vi "PvgeneratorOP500P.vi"(8 "errin":errorcluster, 10 "network":path, 11 "path in":path) -> (0 "sortie d'erreur":errorcluster caption="errout", 1 "network out":path, 2 "tout bon":bool, 3 "Chaîne":string)   [LabVIEW 2020]
uses:
  VG/IS30%_P.vi
  VG/VG_OP400_P.vi
  VG/VG_Conti.vi
  VG/VG_ISOmin_P.vi
  VG/VG_TenmaParam.vi
  VG/VG_OCV30min_P.vi
  VG/VG_OCV30max_P.vi
  VG/VG_OCV70min_P.vi
  VG/VG_OCV70max_P.vi
  VG/VG_DCIRmax_P.vi
  VG/VG_DCIRmin_P.vi
  VG/VG_DCIR+OUIouNON_P.vi
panel:
  out "nombre de remplacements":i32
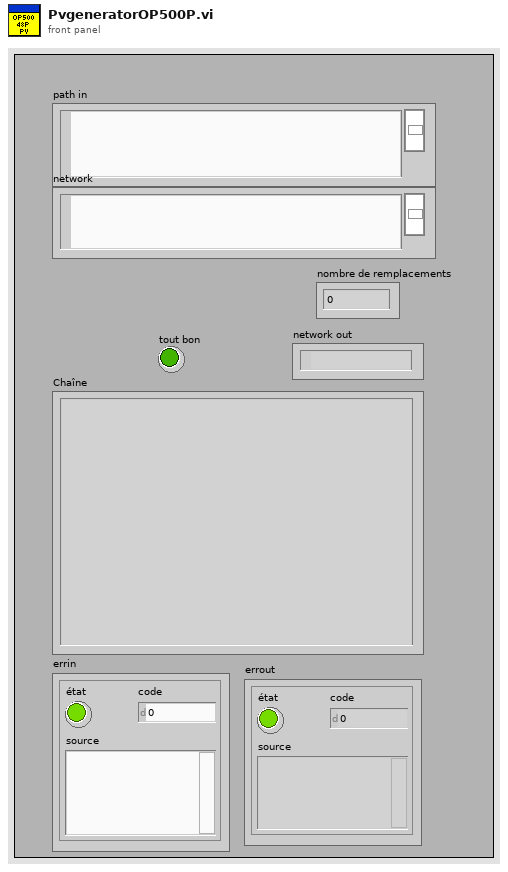
[diagram p1: front panel]
types:
  T1 = enum16{"open", "replace", "create", "open or create", "replace or create", "replace or create with confirmation"}
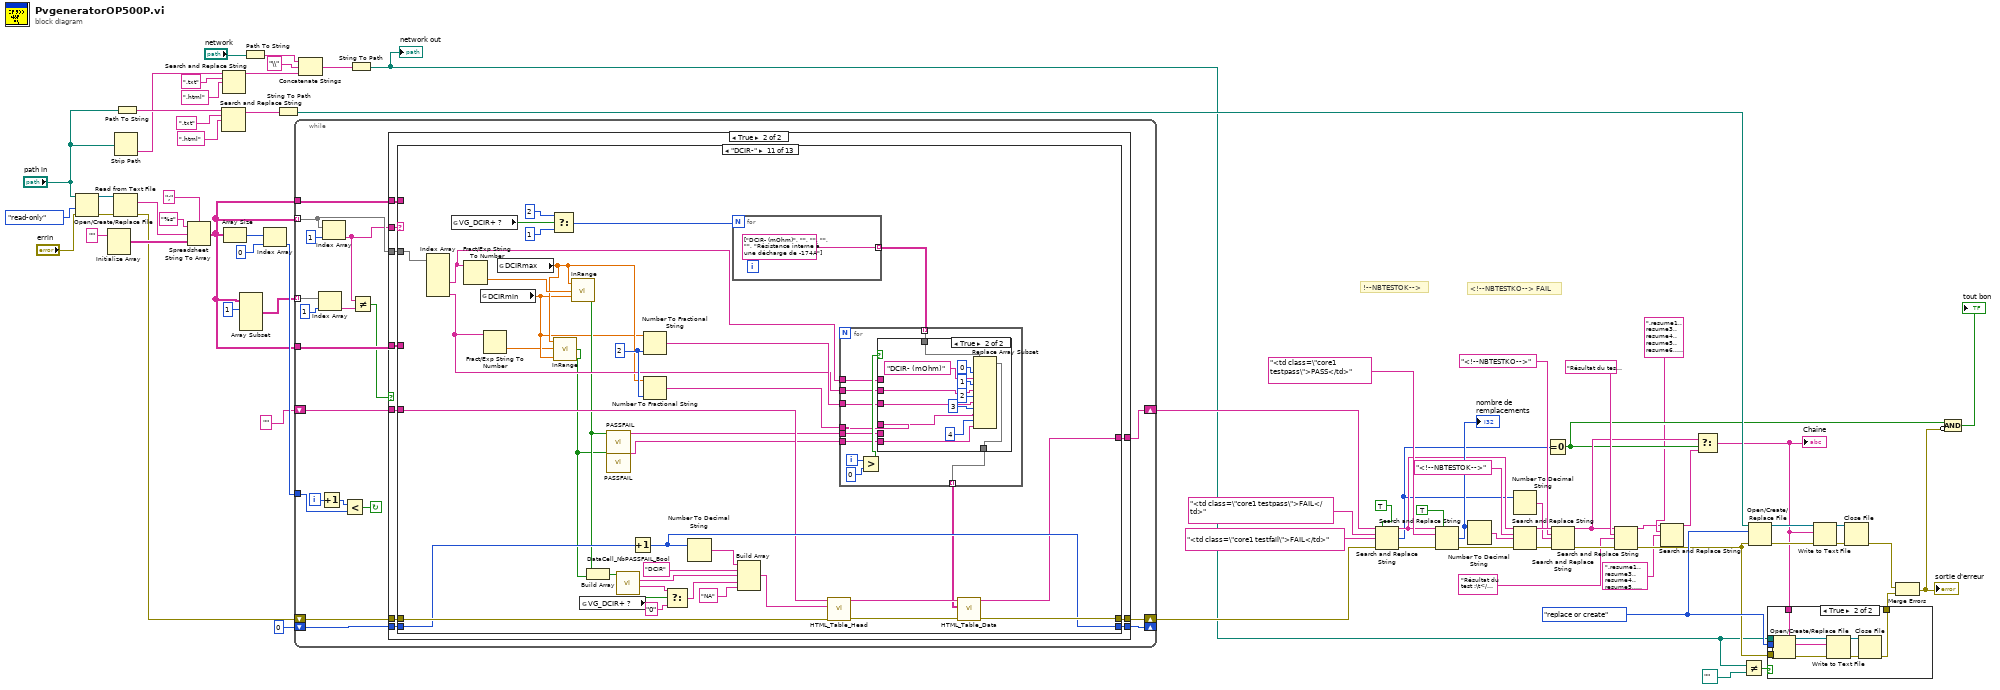
[diagram p0: block diagram]
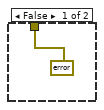
[diagram p2: hidden frame]
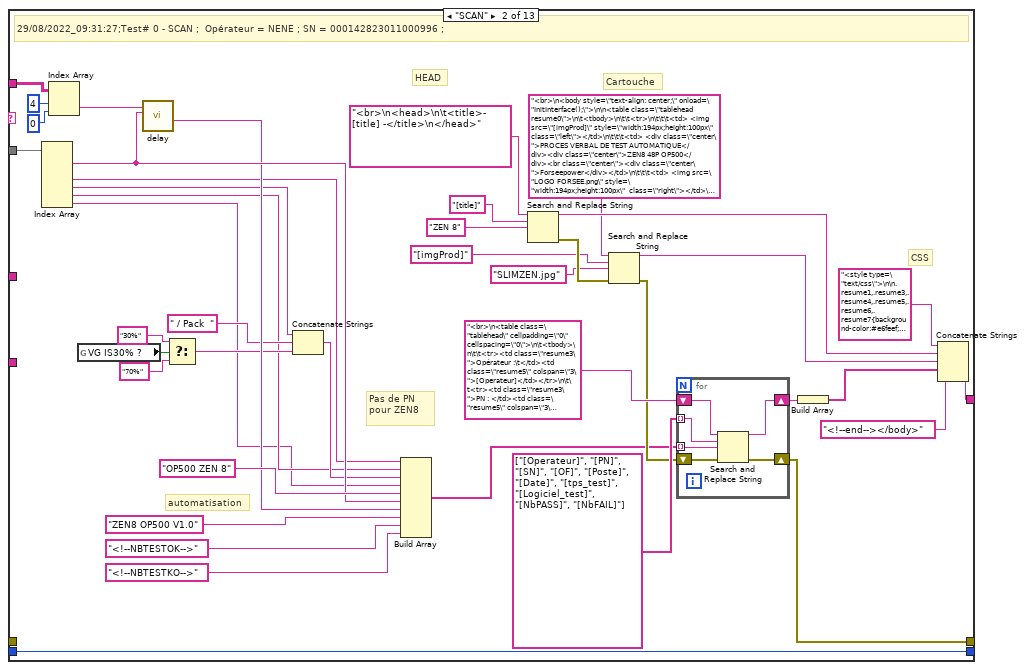
[diagram p5: hidden frame]
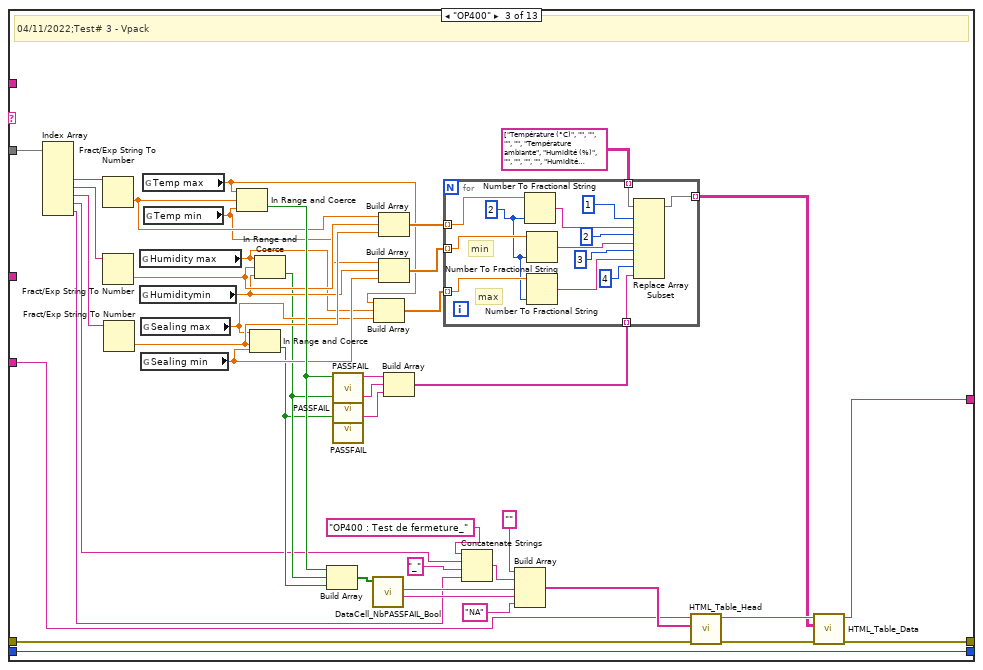
[diagram p6: hidden frame]
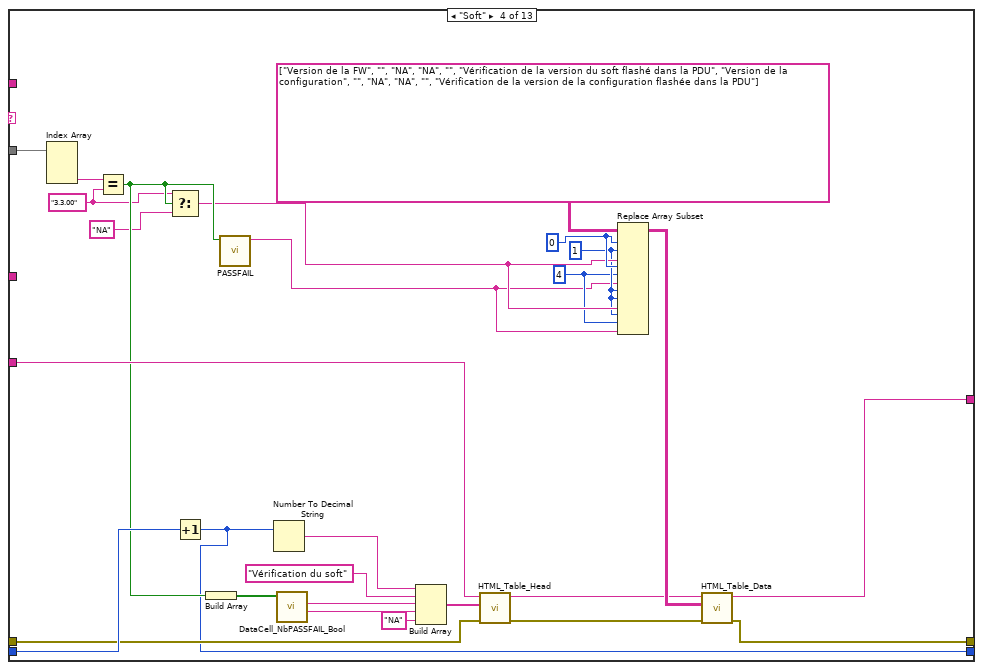
[diagram p7: hidden frame]
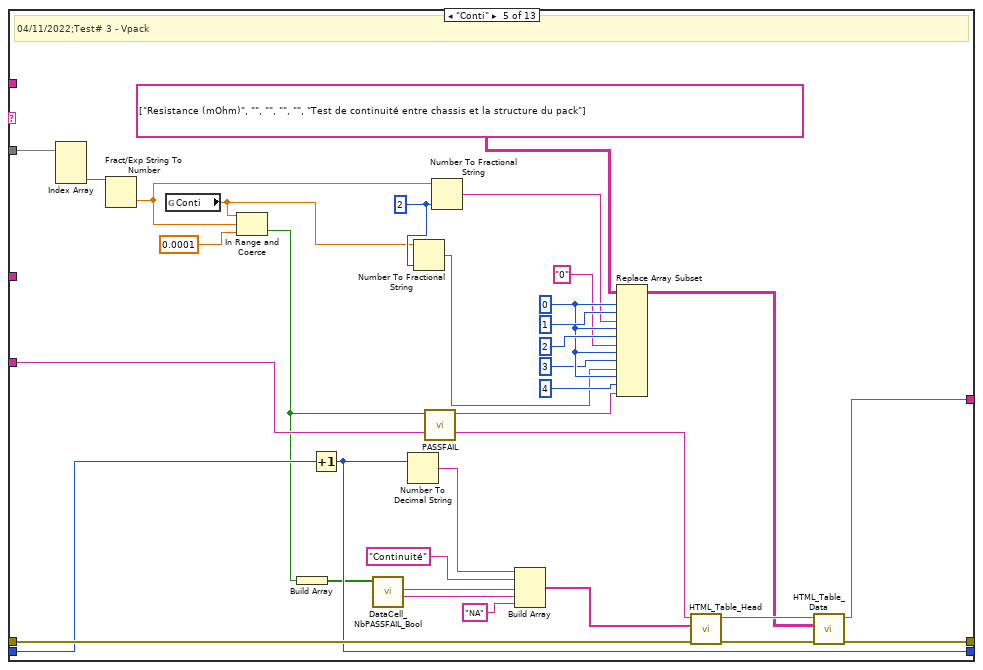
[diagram p8: hidden frame]
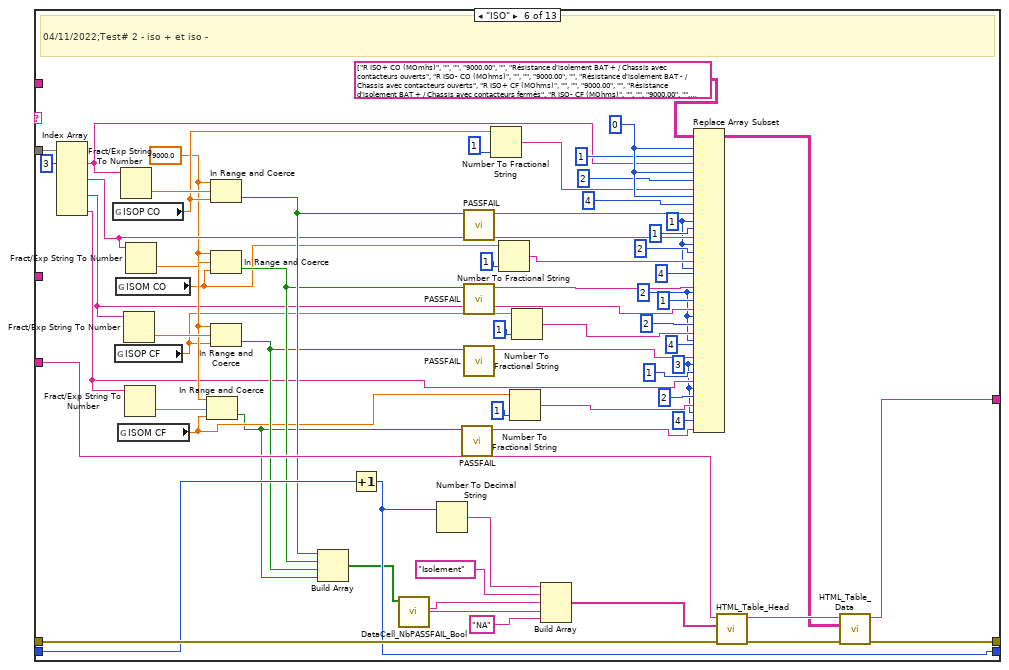
[diagram p9: hidden frame]
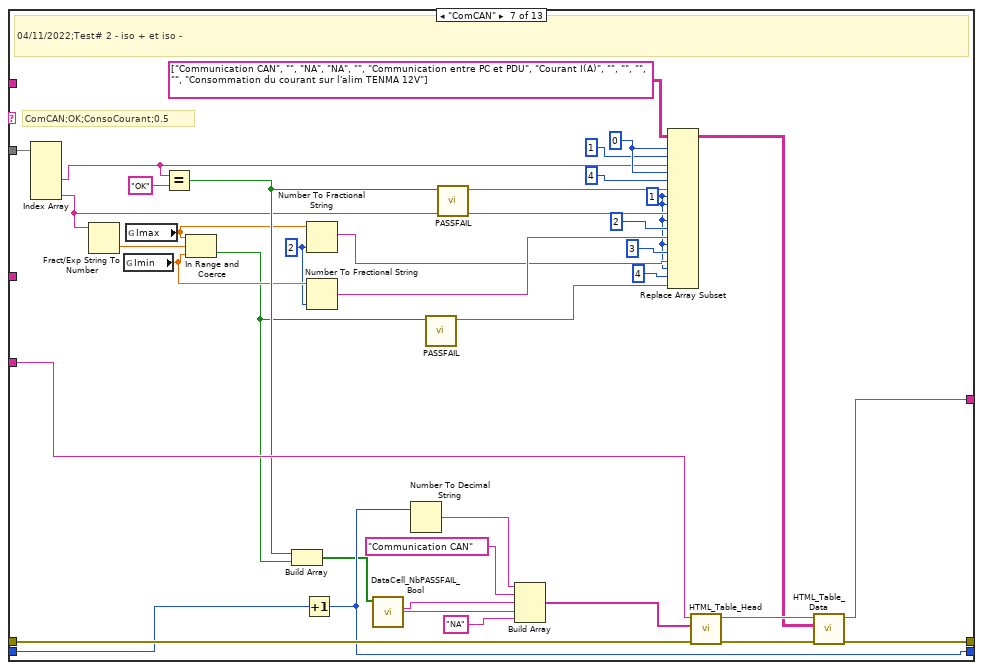
[diagram p10: hidden frame]
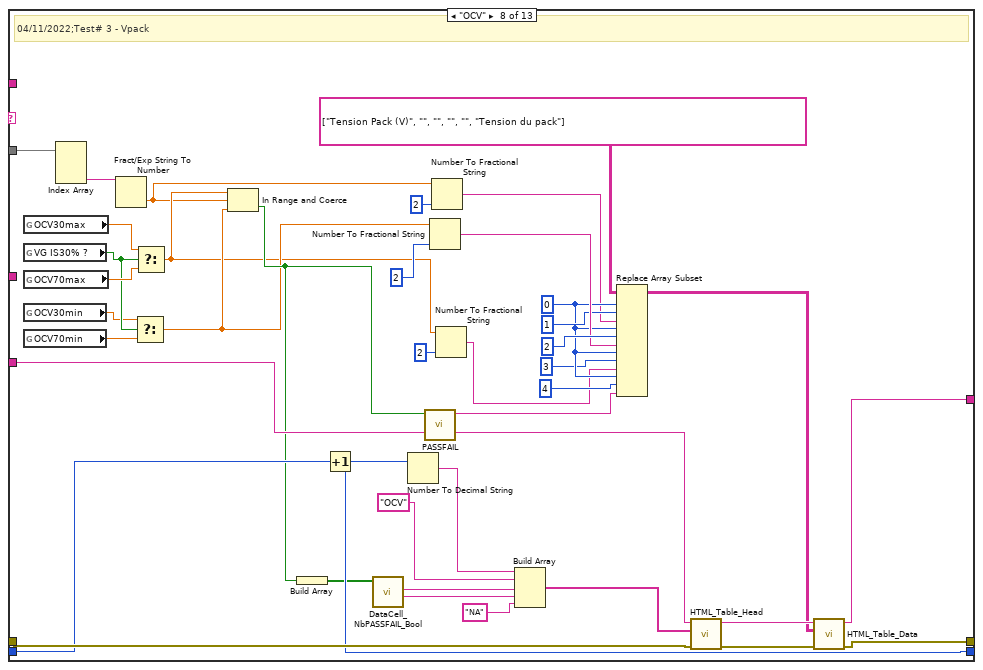
[diagram p11: hidden frame]
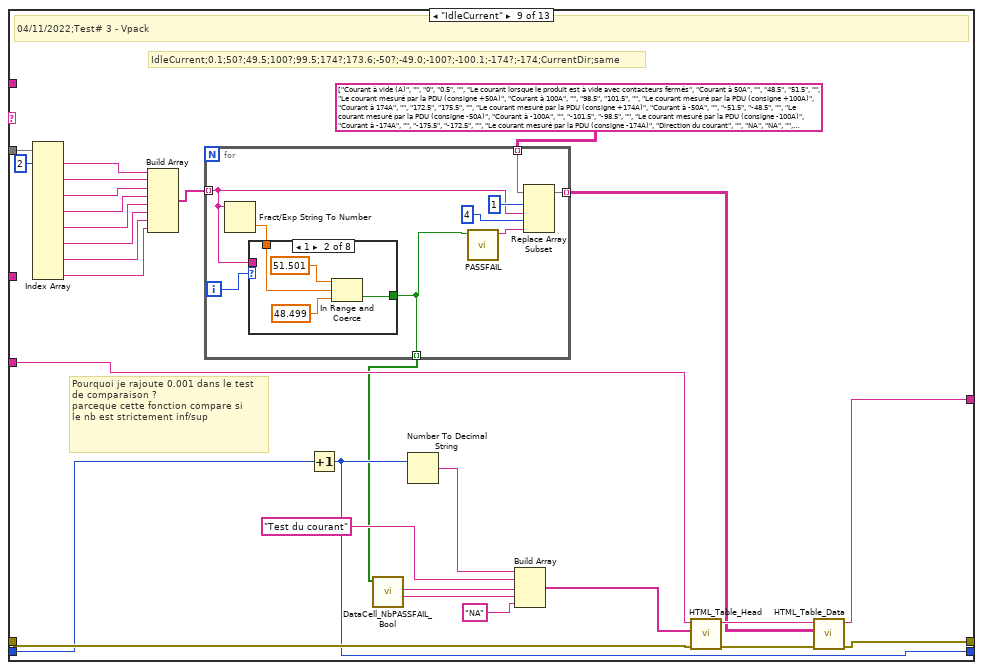
[diagram p12: hidden frame]
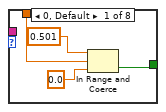
[diagram p13: hidden frame]
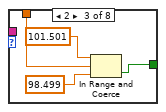
[diagram p14: hidden frame]
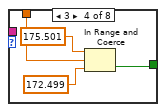
[diagram p15: hidden frame]
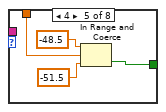
[diagram p16: hidden frame]
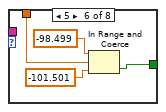
[diagram p17: hidden frame]
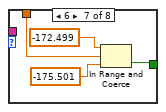
[diagram p18: hidden frame]
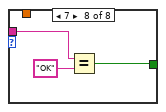
[diagram p19: hidden frame]
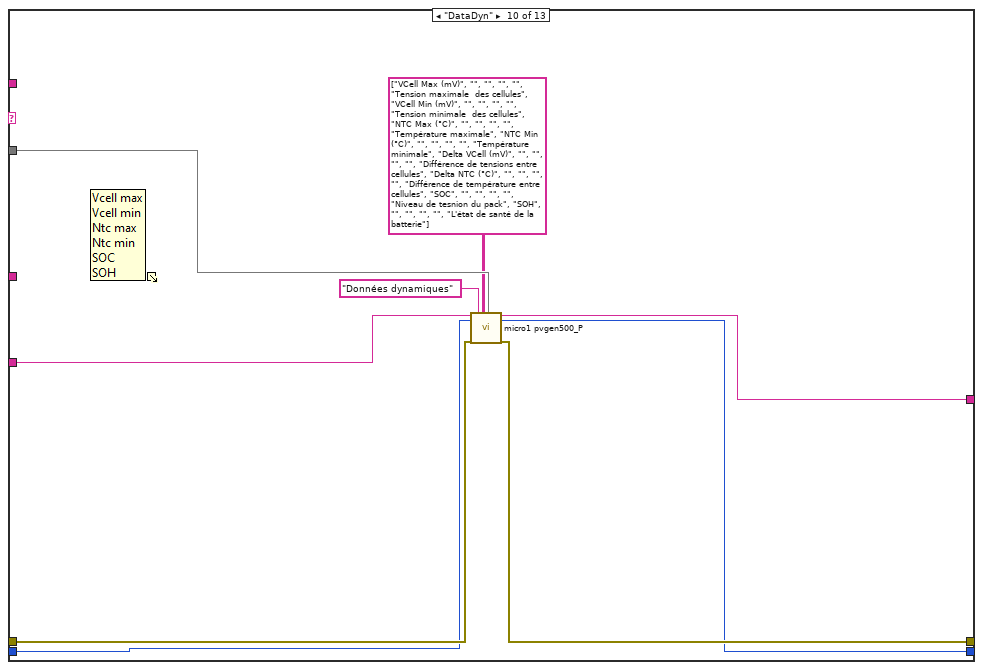
[diagram p20: hidden frame]
diagram:
  w32 = T1."replace or create" ("opération (0 : open)")
  # "<!--NBTESTKO--> FAIL"
  # "!--NBTESTOK-->"
  n1 = Open/Create/Replace File(file path (use dialog)="path in", error in="errin", access (0:read/write)=enum16{"read/write", "read-only", "write-only"}."read-only" ("accès (0 : read/write)")) -> (refnum out=w55:refnum<file>, error out=w72:errorcluster)  [unwired: 3 in, 1 out]
  n2 = Initialize Array("") -> (w70:string[][])  [unwired: 2 in]
  n3 = Read from Text File(file (use dialog)=w55, error in=w72) -> (text=w68:string, error out=w60:errorcluster)  [unwired: 2 in, 2 out]
  n4 = Strip Path(path="path in") -> (name=w13:string)  [unwired: 1 out]
  n5 = Path To String(path="path in") -> (string=w54:string)
  n6 = Spreadsheet String To Array(delimiter (Tab)=";" ("séparateur (Tabulation)"), format string="%s" ("chaîne de format"), spreadsheet string=w68, array type (2D Dbl)=w70) -> (array=w3:string[][])
  n7 = Search and Replace String(input string=w54, search string=".txt" ("chaîne recherchée"), replace string=".html" ("chaîne de remplacement (\"\")")) -> (result string=w51:string)  [unwired: 5 in, 3 out]
  n8 = Search and Replace String(input string=w13, search string=".txt" ("chaîne recherchée"), replace string=".html" ("chaîne de remplacement (\"\")")) -> (result string=w10:string)  [unwired: 5 in, 3 out]
  n9 = Array Size(array=w3) -> (size(s)=w66:i32[])
  n10 = Array Subset(array=w3, index (row)=1 ("indice")) -> (w1:string[][])  [unwired: 3 in]
  n11 = Path To String(path="network") -> (string=w12:string)
  n12 = Index Array(array=w66, index=0 ("indice")) -> (element=w64:i32)
  n13 = String To Path(string=w51) -> (path=w50:path)
  n14 = while {
    tunnel: w64 -> [w91]
    tunnel: w3 -> [w88] mode=indexing
    shift-right: [w87] -> w47
    shift-left: w60 -> [w86]
    shift-right: [w80] -> w49
    shift-left: "" -> [w85]
    shift-right: [w83] -> _
    shift-left: 0 -> [w84]
    tunnel: w3 -> [w82]
    tunnel: w3 -> [w79]
    tunnel: w1 -> [w77] mode=indexing
    i -> [w92]
    stop <- w90 continue-if-true
    n15 = Index Array(array=w77, index=1 ("indice")) -> (element=w76:string)
    n16 = Increment(x=w92) -> (x+1=w81:i32)
    n17 = Index Array(array=w88, index=1 ("indice")) -> (element=w75:string)
    n18 = Less?(x=w81, y=w91) -> (x < y?=w90:bool)
    n19 = Not Equal?(x=w75, y=w76) -> (x != y?=w74:bool)
    n20 = case shown="True" w74 {
      tunnel: w88 -> [_ w105]
      tunnel: [w94 w104] -> w87
      tunnel: w86 -> [w94 w103]
      tunnel: w85 -> [w95 w102]
      tunnel: w84 -> [w93 w101]
      tunnel: [w93 w100] -> w83
      tunnel: w82 -> [_ w99]
      tunnel: [w95 w98] -> w80
      tunnel: w75 -> [_ w97]
      tunnel: w79 -> [_ w96]
      frame False {
      }
      frame True {
        n21 = case shown="\"DCIR-\"" w97 {
          tunnel: w103 -> [w108 _ w192 w234 w264 w328 w366 w406 w435 w491 w525 w589 w618]
          tunnel: w105 -> [_ w149 w193 w228 w265 w329 w367 w407 w436 w487 w528 w579 w608]
          tunnel: [w108 w128 w191 w232 w263 w327 w365 w405 w434 w490 w526 w590 w619] -> w104
          tunnel: w102 -> [w106 _ w190 w238 w262 w326 w364 w404 w433 w485 w519 w580 w609]
          tunnel: w101 -> [w107 w127 w181 w239 w261 w325 w363 w403 w432 w484 w524 w582 w611]
          tunnel: [w107 w127 w181 w214 w260 w324 w362 w402 w431 w483 w521 w564 w603] -> w100
          tunnel: w99 -> [_ _ _ _ _ _ _ _ _ _ _ _ _]
          tunnel: [w106 w126 w189 w216 w259 w323 w361 w401 w430 w489 w512 w578 w607] -> w98
          tunnel: w96 -> [_ w125 _ _ _ _ _ _ _ _ _ _ _]
          frame "NULL", Default {
            # "NULL"
          }
          frame "SCAN" {
            # "automatisation"
            # "Pas de PN pour ZEN8"
            # "Cartouche"
            # "HEAD"
            # "CSS"
            # "29/08/2022_09:31:27;Test# 0 - SCAN ;  Opérateur = NENE ; SN = 000142823011000996 ;"
            n22 = Index Array(array=w149) -> (element #1=w121:string, element #3=w112:string, element #4=w111:string, element #5=w110:string, element #6=w109:string)  [unwired: 6 in, 1 out]
            n23 = Index Array(array=w125, index (row)=4, index (col)=0 ("disabled index (col)")) -> (element=w122:string)
            n24 = global read "IS30%_P.vi" "VG IS30% ?"() -> (w113:bool)
            n25 = call "delay.vi"("String"=w121, "String 2"=w122) -> ("Delay calculé"=w120:string)  [unwired: 9 in]
            n26 = Select(t="30%" ("y"), s=w113, f="70%" ("y")) -> (s? t:f=w116:string)
            n27 = Concatenate Strings(w111, " / Pack  " ("chaîne"), w116) -> (w118:string)
            n28 = Build Array(w112, w110, w118, w109, "OP500 ZEN 8" ("chaîne"), w121, w120, "ZEN8 OP500 V1.0" ("chaîne"), "<!--NBTESTOK-->" ("chaîne"), "<!--NBTESTKO-->" ("chaîne")) -> (w129:string[])
            n29 = Search and Replace String(input string="<br>\n<head>\n\t<title>- [title] -</title>\n</head>", search string="[title]" ("chaîne recherchée"), replace string="ZEN 8" ("Title")) -> (result string=w145:string, error out=w144:errorcluster)  [unwired: 5 in, 2 out]
            n30 = Search and Replace String(input string="<br>\n<body style=\"text-align: center;\" onload=\"InitInterface();\">\n\n<table class=\"tablehead resume0\">\n\t<tbody>\n\t\t<tr>\n\t\t\t<td> <img src=\"[imgProd]\" style=\"width:194px;height:100px\" class=\"left\"></td>\n\t\t\t<td> <div class=\"center\">PROCES VERBAL DE TEST AUTOMATIQUE</div><div class=\"center\">ZEN8 48P OP500</div><br class=\"center\"><div class=\"center\">Forseepower</div></td>\n\t\t\t<td> <img src=\"LOGO FORSEE.png\" style=\"width:194px;height:100px\"  class=\"right\"></td>\n\t\t</tr>\n\t</tbody>\n</table>", search string="[imgProd]", replace string="SLIMZEN.jpg" ("imgProd"), error in=w144) -> (result string=w142:string, error out=w139:errorcluster)  [unwired: 4 in, 2 out]
            n31 = for {
              shift-right: [w154] -> w138
              shift-left: "<br>\n<table class=\"tablehead\" cellpadding=\"0\" cellspacing=\"0\">\n\t<tbody>\n\t\t<tr><td class=\"resume3\">Opérateur :\t</td><td class=\"resume5\" colspan=\"3\">[Operateur]</td></tr>\n\t\t<tr><td class=\"resume3\">PN : </td><td class=\"resume5\" colspan=\"3\">[PN]</td></tr>\n\t\t<tr><td class=\"resume3\">SN : </td><td class=\"resume5\" colspan=\"3\">[SN]</td></tr>\n\t\t<tr><td class=\"resume3\">OF : </td><td class=\"resume5\" colspan=\"3\">[OF]</td></tr>\n\t\t<tr><td class=\"resume3\">Poste : </td><td class=\"resume5\" colspan=\"3\">[Poste]</td></tr>\t\t\n\t\t<tr><td class=\"resume3\">Date du test : </td><td class=\"resume5\" colspan=\"3\">[Date]</td></tr>\n\t\t<tr><td class=\"resume3\">Temps de test : </td><td class=\"resume5\" colspan=\"3\">[tps_test]</td></tr>\n\t\t<tr><td class=\"resume3\">Logiciel de test :\t</td><td class=\"resume5\" colspan=\"3\">[Logiciel_test]</td></tr>\n\t\t<tr><td class=\"resume3\">Résultat du test :\t</td><td class=\"resume5\" colspan=\"3\"><div><span style=\"float:left\" id=\"result\"><font size = \"5pt\" color=\"green\"><b>CONFORME</b></font><b><font size = \"5pt\"> ( </font><font size = \"5pt\" color=\"green\">[NbPASS] PASS </font>  <font size = \"5pt\"> / </font><font size = \"5pt\" color=\"red\">[NbFAIL] FAIL</font> <font size = \"5pt\"> ) </font></b></span></div></td></tr>\n\t</tbody>\n</table>" -> [w155]
              tunnel: string[] ["[Operateur]", "[PN]", "[SN]", "[OF]", "[Poste]", "[Date]", "[tps_test]", "[Logiciel_test]", "[NbPASS]", "[NbFAIL]"] -> [w151] mode=indexing
              tunnel: w129 -> [w150] mode=indexing
              shift-right: [w152] -> w128
              shift-left: w139 -> [w153]
              n32 = Search and Replace String(input string=w155, search string=w151, replace string=w150, error in=w153) -> (result string=w154:string, error out=w152:errorcluster)  [unwired: 4 in, 2 out]
            }
            n33 = Build Array(w138) -> (w137:string[])
            n34 = Concatenate Strings("<style type=\"text/css\">\n\n.resume1,.resume3,.resume4,.resume5,.resume6,.resume7{background-color:#e6feef;padding:7px;border:1px solid black;}\n.resume0{border:1px solid black;background-color:#e6feef;font-weight: bold;padding:0px;text-align: center;}\n.resume1{width:350px;text-align:right;font-weight:bold;}\n.resume3{width:350px;text-align:right;border-top:0px solid black;font-weight:bold;}\n.resume4{border-left:0px solid black;width:290px;}\n.resume5{width:290px;border-left:0px solid black;border-top:0px solid black;}\n.resume6{border-left:0px solid black;width:60px;}\n.resume7{border-left:0px solid black;border-top:0px solid black;width:60px;}\n.title1{text-align: left;background-color:#e6f4fe;padding:10px;border:1px solid #101010;}\n.title2{width: 30px;text-align: center;background-color:#e6f4fe;padding:1px;border:1px solid #101010;border-left:0px solid black;font-weight: bold;}\n.title2 a:link{text-decoration:none;}\n.entete0,.entete1,.entete2,.time2{text-align: center;background-color:#feeec9;padding:7px;border:1px solid black;font-weight: bold;}\n.entete0{width:45px;border-right:0px solid black;}\n.entete1{width:505px;}\n.entete2{width:95px;border-right:0px solid black;}\n.time2{border-left:0px solid black;width:145px;font-size:11px;}\n.core0,.core1,.core2,.core3,.core4,.time{text-align: center;background-color:#fafed3;padding:7px;border:1px solid black;}\n.core0, .core1,.core3,.core4{width:95px;border-top:0px solid black;border-right:0px solid black;}\n.core0{width:45px;}\n.core2{border-top:0px solid black;width:505px;}\n.core3{width:200px;}\n.core4{width:300px;}\n.time{width:145px;border-top:0px solid black;border-left:0px solid black;font-size:11px;}\n.false .core0,.false .core1,.false .core2,.false .core3,.false .core4,.false .time{background-color:#f4f4f4;}\n.false .entete0,.false .entete1,.false .entete2,.false .time2{background-color:#dadada;}\n.false .title1,.false .title2,.false .resultentete .testpass,.false .resultentete .testfail,.false .resultentete .testtime{background-color:#c5cac9;color: blue;}\n.false .title2 a:link{text-decoration:none;color: blue;}\n.comment1,.comment2,.time3{width: 890px;background-color:#e9e8e9;padding:7px;border:1px solid black;border-top:0px solid black;text-align:left;}\n.comment2{border-right:0px solid black;width: 45px;text-align: center;}\n.time3{width: 145px;border-left:0px solid black;font-size:11px;}\n.fixe1{background: -moz-linear-gradient(center top , #101010 10%, #555555 80%) repeat scroll 0 0 transparent;background: -webkit-gradient(linear, left top, left bottom, from(#101010), to(#555555));border:2px solid orange;position : fixed;margin-top:20px;display:none;overflow-y:scroll;max-height:350px;text-shadow: 0px 0px 0 #333333;text-align:left;font-size:10px;padding:10px;margin-left:-162px;border-radius: 15px 15px 15px 15px;}\n.menufixe, .menufixelock{background: -moz-linear-gradient(center top , #101010 80%, transparent 20%) repeat scroll 0 0 transparent;background: -webkit-gradient(linear, left top, left bottom, from(#101010), color-stop(0.65, #101010), to(transparent)) repeat scroll 0 0 transparent;margin: -52px 0px 0px -9px;width:100%;position:fixed;height:55px;-moz-transition: margin 1s;-webkit-transition: margin 1s;}\n.menufixelock, .menufixe:hover{margin: -9px 0px 0px -9px;}\n.lockmenu, .separation,.separationmenu{text-align:center;background: -moz-linear-gradient(center top , #555555 10%, #111111 80%) repeat scroll 0 0 transparent;background: -webkit-gradient(linear, left top, left bottom, from(#555555), to(#111111));border: 1px solid white;border-radius: 10px 10px 10px 10px;box-shadow: 0 -1px 1px #555555 inset;color: #999999;font-weight: bold;width: 100px;padding: 2px;text-decoration: none;}\n.tablehead{width: 1000px;font-family: Verdana;font-size: 12px;margin-left: auto;margin-right: auto;}\n.tablenull{font-family: Verdana;font-size: 11px;margin-left: auto;margin-right: auto;}\n.separationmenu:hover div{display: inline;}\n.lockmenu:hover, .separation:hover,.separationmenu:hover{border: 1px solid orange;cursor:pointer;}\n.lockmenu:hover{border: 1px solid red;cursor:pointer;}\n.separationright{padding:10px;}\ndiv a:link{text-decoration:none;color:#cbcbcb;}\ndiv a:hover{text-decoration:underline;color:#cbcbcb;}\nspan a:link{text-decoration:none;color:#cbcbcb;}\nspan a:hover{text-decoration:none;color:#cbcbcb;}\n.false{color: blue;}\n.testpass{color: green;font-weight: bold;}\n.testfail{color: red;font-weight: bold;}\n.testtime{color: blue;font-weight: bold;}\n.resultentete{font-weight: bold;font-size: 11px;min-width: 200px;text-align:right;}\n.infohard{border: 1px solid black;background-color: white;text-align: center;width: 16px;height: 16px;border-radius: 5px;font-weight: bold;box-shadow: 0 -1px 2px #555555 inset;}\n.infohard:hover{background-color:#feeec9;cursor:pointer;}\n.footerhard{padding-top:30px;}\n.confighard{font-size:10px;width:110px;}\n.circlemain{margin-left:auto;margin-right:auto;}\n.circletext,.circleform{padding-top: 3px;text-align:center;font-size: 10px;width:200px;}\n.circleform{padding-bottom: 3px;padding-top: 1px;}\n.circle{border: 1px solid black;border-collapse: collapse;border-radius: 15px;box-shadow: 1px 1px 0 #505050;height: 15px;width: 15px;display:inline-block;}\n.bookmarkon, .bookmarkoff{background-color: yellow;border: 1px solid black;border-collapse: collapse;border-radius: 10px 10px 10px 10px;box-shadow: 1px 1px 0 #505050;height: 12px;width: 12px;position: absolute;margin-left:22px;cursor: help;}\n.bookmarkoff{background-color: transparent;border: 1px solid #CECECE;box-shadow: none;cursor: copy;}\n.false .bookmarkoff{background-color: transparent;border: 1px solid #E6E1E1;box-shadow: none;cursor: copy;}\n.bookmarkmaster{height: 15px;margin-right: 12px;width: 60px;}\n.bookmarkmaster:hover .bookmarkprev,.bookmarkmaster:hover .bookmarksuiv{display:block;}\n.bookmarkprev, .bookmarksuiv {cursor: pointer;font-size: 25px;font-weight: bold;margin-top: -10px;position: absolute;display:none;}\n.bookmarkprev{margin-left: 2px;}\n.bookmarksuiv{margin-left: 43px;}\n.plus, .moins{background-color: #F4F4F4;border: 1px solid #848484;border-radius: 20px;color: #848484;font-family: arial;font-size: 16px;font-weight: bold;height: 20px;margin-left: 4px;text-align: center;width: 20px;}\n.moins{font-size: 15px;}\n.plus:hover, .moins:hover{background-color: #DADADA;border: 1px solid black;color: black;cursor:pointer;}\n.backtothetop {position: fixed; right: 50%; margin-right: -555px; bottom: 10px; font-size: 35px; font-weight: bold; border: 1px solid #7D7B91; width: 40px; height: 40px; line-height:52px; text-align: center;border-radius: 8px; opacity: 0.25; background-color: #F5F5F5; color:#7D7B91;}\n.backtothetop:hover {opacity: 1; cursor:pointer;}\n.libversion {font-size: 8px;font-weight: normal;padding-right: 10px;text-align: right;}\n.lockmenu {width: 18px;font-size: 12px;}\n.left {display: block; margin-left: 1px;margin-right: auto;}\n.right {display: block; margin-right: 1px;margin-left: auto;}\n.center {display: block; margin-left: auto;margin-right: auto;}\n\n</style>", w145, w142, w137, "<!--end--></body>") -> (w126:string)
          }
          frame "OP400" {
            # "04/11/2022;Test# 3 - Vpack"
            n35 = Index Array(array=w193) -> (element #3=w184:string, element #4=w180:string, element #5=w179:string, element #6=w158:string, element #7=w156:string)  [unwired: 7 in, 2 out]
            n36 = Fract/Exp String To Number(string=w184) -> (number=w178:dbl)  [unwired: 3 in, 1 out]
            n37 = Fract/Exp String To Number(string=w180) -> (number=w177:dbl)  [unwired: 3 in, 1 out]
            n38 = Fract/Exp String To Number(string=w179) -> (number=w176:dbl)  [unwired: 3 in, 1 out]
            n39 = global read "VG_OP400_P.vi" "Humidity max"() -> (w169:dbl)
            n40 = global read "VG_OP400_P.vi" "Humiditymin"() -> (w173:dbl)
            n41 = global read "VG_OP400_P.vi" "Sealing max"() -> (w168:dbl)
            n42 = global read "VG_OP400_P.vi" "Sealing min"() -> (w172:dbl)
            n43 = global read "VG_OP400_P.vi" "Temp max"() -> (w170:dbl)
            n44 = global read "VG_OP400_P.vi" "Temp min"() -> (w174:dbl)
            n45 = In Range and Coerce(upper limit=w170, x=w178, lower limit=w174) -> (In Range?=w183:bool)  [unwired: 1 out]
            n46 = In Range and Coerce(upper limit=w168, x=w176, lower limit=w172) -> (In Range?=w164:bool)  [unwired: 1 out]
            n47 = In Range and Coerce(upper limit=w169, x=w177, lower limit=w173) -> (In Range?=w165:bool)  [unwired: 1 out]
            n48 = Build Array(w183, w165, w164) -> (w187:bool[])
            n49 = call <userlib>:"PASSFAIL.vi"("E"=w183) -> ("S"=w166:string)  [unwired: 10 in]
            n50 = call <userlib>:"PASSFAIL.vi"("E"=w165) -> ("S"=w163:string)  [unwired: 10 in]
            n51 = call <userlib>:"PASSFAIL.vi"("E"=w164) -> ("S"=w162:string)  [unwired: 10 in]
            n52 = call <userlib>:"DataCell_NbPASSFAIL_Bool.vi"("Tableau en entrée"=w187) -> ("Chaîne"=w185:string, "Chaîne 2"=w186:string)  [unwired: 8 in, 1 out]
            n53 = Build Array(w170, w169, w168) -> (w167:dbl[])
            n54 = Build Array(w178, w177, w176) -> (w175:dbl[])
            n55 = Build Array(w174, w173, w172) -> (w171:dbl[])
            n56 = Build Array(w166, w163, w162) -> (w161:string[])
            n57 = for {
              tunnel: string[][] [["Température (°C)", "", "", "", "", "Température ambiante"], ["Humidité (%)", "", "", "", "", "Humidité ambiante"], ["Etanchéité (Pa)", "", "", "", "", "Etanchéité du pack"]] ("Tableau") -> [w212] mode=indexing
              tunnel: [w208] -> w188 mode=indexing
              tunnel: w175 -> [w207] mode=indexing
              tunnel: w171 -> [w204] mode=indexing
              tunnel: w167 -> [w203] mode=indexing
              tunnel: w161 -> [w199] mode=indexing
              w202 = i16 2 ("précision (6)")
              # "max"
              # "min"
              n58 = Number To Fractional String(number=w207, precision (6)=w202) -> (F-format string=w209:string)  [unwired: 2 in]
              n59 = Number To Fractional String(number=w204, precision (6)=w202) -> (F-format string=w210:string)  [unwired: 2 in]
              n60 = Number To Fractional String(number=w203, precision (6)=w202) -> (F-format string=w201:string)  [unwired: 2 in]
              n61 = Replace Array Subset(array=w212, new element #1=w209, index #1=1 ("index"), new element #2=w210, index #2=2 ("index"), new element #3=w201, index #3=3 ("index"), new element #4=w199, index #4=4 ("index")) -> (w208:string[])
            }
            n62 = Concatenate Strings("OP400 : Test de fermeture_" ("élément"), w158, "_" ("string"), w156) -> (w159:string)
            n63 = Build Array("" ("element"), w159, w186, w185, "NA" ("élément")) -> (w197:string[])
            n64 = call "HTML_Table_Head.vi"("entrée d'erreur (pas d'erreur)"=w192, "Tableau"=w197, "chaîne en entrée"=w190) -> ("sortie d'erreur"=w196:errorcluster, "result string"=w195:string)  [unwired: 7 in]
            n65 = call "HTML_Table_Data.vi"("entrée d'erreur (pas d'erreur)"=w196, "Tableau"=w188, "chaîne en entrée"=w195) -> ("sortie d'erreur"=w191:errorcluster, "result string"=w189:string)  [unwired: 7 in]
          }
          frame "Soft" {
            w220 = 4 ("disabled index (col)")
            w223 = 0 ("disabled index (row)")
            w224 = "3.3.00" ("y")
            w221 = 1 ("disabled index (col)")
            n66 = Index Array(array=w228) -> (element #3=w227:string)  [unwired: 3 in, 2 out]
            n67 = Equal?(x=w227, y=w224) -> (x = y?=w225:bool)
            n68 = Select(t=w224, s=w225, f="NA") -> (s? t:f=w222:string)
            n69 = Increment(x=w239) -> (x+1=w214:i32)
            n70 = Build Array(w225) -> (w226:bool[])
            n71 = call <userlib>:"PASSFAIL.vi"("E"=w225) -> ("S"=w219:string)  [unwired: 10 in]
            n72 = Number To Decimal String(number=w214) -> (decimal integer string=w236:string)  [unwired: 1 in]
            n73 = call <userlib>:"DataCell_NbPASSFAIL_Bool.vi"("Tableau en entrée"=w226) -> ("Chaîne"=w230:string, "Chaîne 2"=w231:string)  [unwired: 8 in, 1 out]
            n74 = Build Array(w236, "Vérification du soft" ("element"), w231, w230, "NA" ("element")) -> (w237:string[])
            n75 = call "HTML_Table_Head.vi"("entrée d'erreur (pas d'erreur)"=w234, "Tableau"=w237, "chaîne en entrée"=w238) -> ("sortie d'erreur"=w233:errorcluster, "result string"=w217:string)  [unwired: 7 in]
            n76 = Replace Array Subset(array=string[][] [["Version de la FW", "", "NA", "NA", "", "Vérification de la version du soft flashé dans la PDU"], ["Version de la configuration", "", "NA", "NA", "", "Vérification de la version de la configuration flashée dans la PDU"]] ("Tableau"), new element #1=w222, index (row) #1=w223, index (col) #1=w221, new element #2=w219, index (row) #2=w223, index (col) #2=w220, new element #3=w222, index (row) #3=w221, index (col) #3=w221, new element #4=w219, index (row) #4=w221, index (col) #4=w220) -> (w218:string[][])
            n77 = call "HTML_Table_Data.vi"("entrée d'erreur (pas d'erreur)"=w233, "Tableau"=w218, "chaîne en entrée"=w217) -> ("sortie d'erreur"=w232:errorcluster, "result string"=w216:string)  [unwired: 7 in]
          }
          frame "Conti" {
            w242 = i16 2 ("précision (6)")
            w249 = 0 ("index (row)")
            # "04/11/2022;Test# 3 - Vpack"
            n78 = Index Array(array=w265) -> (element #3=w252:string)  [unwired: 3 in, 2 out]
            n79 = Fract/Exp String To Number(string=w252) -> (number=w246:dbl)  [unwired: 3 in, 1 out]
            n80 = global read "VG_Conti.vi" "Conti"() -> (w241:dbl)
            n81 = In Range and Coerce(upper limit=w241, x=w246, lower limit=0.0001) -> (In Range?=w247:bool)  [unwired: 1 out]
            n82 = Build Array(w247) -> (w257:bool[])
            n83 = Increment(x=w261) -> (x+1=w260:i32)
            n84 = call <userlib>:"DataCell_NbPASSFAIL_Bool.vi"("Tableau en entrée"=w257) -> ("Chaîne"=w255:string, "Chaîne 2"=w256:string)  [unwired: 8 in, 1 out]
            n85 = Number To Decimal String(number=w260) -> (decimal integer string=w268:string)  [unwired: 1 in]
            n86 = Number To Fractional String(number=w241, precision (6)=w242) -> (F-format string=w240:string)  [unwired: 2 in]
            n87 = call <userlib>:"PASSFAIL.vi"("E"=w247) -> ("S"=w251:string)  [unwired: 10 in]
            n88 = Number To Fractional String(number=w246, precision (6)=w242) -> (F-format string=w245:string)  [unwired: 2 in]
            n89 = Build Array(w268, "Continuité" ("élément"), w256, w255, "NA" ("élément")) -> (w271:string[])
            n90 = Replace Array Subset(array=string[][] [["Resistance (mOhm)", "", "", "", "", "Test de continuité entre chassis et la structure du pack"]] ("Tableau"), new element #1=w245, index (row) #1=w249, index (col) #1=1 ("disabled index (col)"), new element #2="0" ("new element/subarray"), index (row) #2=w249, index (col) #2=2 ("disabled index (col)"), new element #3=w240, index (row) #3=w249, index (col) #3=3 ("disabled index (col)"), new element #4=w251, index (row) #4=w249, index (col) #4=4 ("disabled index (col)")) -> (w258:string[][])
            n91 = call "HTML_Table_Head.vi"("entrée d'erreur (pas d'erreur)"=w264, "Tableau"=w271, "chaîne en entrée"=w262) -> ("sortie d'erreur"=w270:errorcluster, "result string"=w269:string)  [unwired: 7 in]
            n92 = call "HTML_Table_Data.vi"("entrée d'erreur (pas d'erreur)"=w270, "Tableau"=w258, "chaîne en entrée"=w269) -> ("sortie d'erreur"=w263:errorcluster, "result string"=w259:string)  [unwired: 7 in]
          }
          frame "ISO" {
            w276 = 3 ("index (row)")
            w284 = 2 ("index (row)")
            w294 = 1 ("index (row)")
            w299 = 9000.0 ("limite supérieure")
            w317 = 0 ("index (row)")
            # "04/11/2022;Test# 2 - iso + et iso -"
            n93 = Index Array(array=w329, index #1=3 ("index")) -> (element #1=w305:string, element #3=w303:string, element #5=w290:string, element #7=w281:string)  [unwired: 6 in, 3 out]
            n94 = global read "VG_ISOmin_P.vi" "ISOP CO"() -> (w307:dbl)
            n95 = global read "VG_ISOmin_P.vi" "ISOP CF"() -> (w288:dbl)
            n96 = global read "VG_ISOmin_P.vi" "ISOM CO"() -> (w296:dbl)
            n97 = global read "VG_ISOmin_P.vi" "ISOM CF"() -> (w278:dbl)
            n98 = Fract/Exp String To Number(string=w305) -> (number=w311:dbl)  [unwired: 3 in, 1 out]
            n99 = Fract/Exp String To Number(string=w290) -> (number=w302:dbl)  [unwired: 3 in, 1 out]
            n100 = Fract/Exp String To Number(string=w281) -> (number=w300:dbl)  [unwired: 3 in, 1 out]
            n101 = Fract/Exp String To Number(string=w303) -> (number=w308:dbl)  [unwired: 3 in, 1 out]
            n102 = In Range and Coerce(upper limit=w299, x=w300, lower limit=w278) -> (In Range?=w273:bool)  [unwired: 1 out]
            n103 = In Range and Coerce(upper limit=w299, x=w311, lower limit=w307) -> (In Range?=w310:bool)  [unwired: 1 out]
            n104 = In Range and Coerce(upper limit=w299, x=w308, lower limit=w296) -> (In Range?=w309:bool)  [unwired: 1 out]
            n105 = In Range and Coerce(upper limit=w299, x=w302, lower limit=w288) -> (In Range?=w301:bool)  [unwired: 1 out]
            n106 = Build Array(w310, w309, w301, w273) -> (w321:bool[])
            n107 = Increment(x=w325) -> (x+1=w324:i32)
            n108 = call <userlib>:"DataCell_NbPASSFAIL_Bool.vi"("Tableau en entrée"=w321) -> ("Chaîne"=w319:string, "Chaîne 2"=w320:string)  [unwired: 8 in, 1 out]
            n109 = Number To Decimal String(number=w324) -> (decimal integer string=w332:string)  [unwired: 1 in]
            n110 = call <userlib>:"PASSFAIL.vi"("E"=w273) -> ("S"=w274:string)  [unwired: 10 in]
            n111 = call <userlib>:"PASSFAIL.vi"("E"=w310) -> ("S"=w316:string)  [unwired: 10 in]
            n112 = call <userlib>:"PASSFAIL.vi"("E"=w309) -> ("S"=w292:string)  [unwired: 10 in]
            n113 = call <userlib>:"PASSFAIL.vi"("E"=w301) -> ("S"=w283:string)  [unwired: 10 in]
            n114 = Number To Fractional String(number=w307, precision (6)=i16 1) -> (F-format string=w312:string)  [unwired: 2 in]
            n115 = Number To Fractional String(number=w296, precision (6)=i16 1) -> (F-format string=w295:string)  [unwired: 2 in]
            n116 = Number To Fractional String(number=w278, precision (6)=i16 1) -> (F-format string=w277:string)  [unwired: 2 in]
            n117 = Number To Fractional String(number=w288, precision (6)=i16 1) -> (F-format string=w287:string)  [unwired: 2 in]
            n118 = Build Array(w332, "Isolement" ("élément"), w320, w319, "NA" ("élément")) -> (w335:string[])
            n119 = Replace Array Subset(array=string[][] [["R ISO+ CO (MOmhs)", "", "", "9000.00", "", "Résistance d'isolement BAT + / Chassis avec contacteurs ouverts"], ["R ISO- CO (MOhms)", "", "", "9000.00", "", "Résistance d'isolement BAT - / Chassis avec contacteurs ouverts"], ["R ISO+ CF (MOhms)", "", "", "9000.00", "", "Résistance d'isolement BAT + / Chassis avec contacteurs fermés"], ["R ISO- CF (MOhms)", "", "", "9000.00", "", "Résistance d'isolement BAT - / Chassis avec contacteurs fermés"]] ("Tableau"), new element #1=w305, index (row) #1=w317, index (col) #1=1 ("disabled index (col)"), new element #2=w312, index (row) #2=w317, index (col) #2=2 ("disabled index (col)"), new element #3=w316, index (row) #3=w317, index (col) #3=4 ("disabled index (col)"), new element #4=w303, index (row) #4=w294, index (col) #4=1 ("disabled index (col)"), new element #5=w295, index (row) #5=w294, index (col) #5=2 ("disabled index (col)"), new element #6=w292, index (row) #6=w294, index (col) #6=4 ("disabled index (col)"), new element #7=w290, index (row) #7=w284, index (col) #7=1 ("disabled index (col)"), new element #8=w287, index (row) #8=w284, index (col) #8=2 ("disabled index (col)"), new element #9=w283, index (row) #9=w284, index (col) #9=4 ("index (row)"), new element #10=w281, index (row) #10=w276, index (col) #10=1 ("disabled index (col)"), new element #11=w277, index (row) #11=w276, index (col) #11=2 ("disabled index (col)"), new element #12=w274, index (row) #12=w276, index (col) #12=4 ("disabled index (col)")) -> (w322:string[][])
            n120 = call "HTML_Table_Head.vi"("entrée d'erreur (pas d'erreur)"=w328, "Tableau"=w335, "chaîne en entrée"=w326) -> ("sortie d'erreur"=w334:errorcluster, "result string"=w333:string)  [unwired: 7 in]
            n121 = call "HTML_Table_Data.vi"("entrée d'erreur (pas d'erreur)"=w334, "Tableau"=w322, "chaîne en entrée"=w333) -> ("sortie d'erreur"=w327:errorcluster, "result string"=w323:string)  [unwired: 7 in]
          }
          frame "ComCAN" {
            w337 = i16 2 ("precision (6)")
            w340 = 1 ("index (row)")
            w356 = 0 ("index (row)")
            # "ComCAN;OK;ConsoCourant;0.5"
            # "04/11/2022;Test# 2 - iso + et iso -"
            n122 = Index Array(array=w367) -> (element #3=w351:string, element #5=w348:string)  [unwired: 5 in, 3 out]
            n123 = Fract/Exp String To Number(string=w348) -> (number=w353:dbl)  [unwired: 3 in, 1 out]
            n124 = global read "VG_TenmaParam.vi" "Imin"() -> (w346:dbl)
            n125 = global read "VG_TenmaParam.vi" "Imax"() -> (w347:dbl)
            n126 = Equal?(x=w351, y="OK") -> (x = y?=w349:bool)
            n127 = In Range and Coerce(upper limit=w347, x=w353, lower limit=w346) -> (In Range?=w341:bool)  [unwired: 1 out]
            n128 = Build Array(w349, w341) -> (w359:bool[])
            n129 = Increment(x=w363) -> (x+1=w362:i32)
            n130 = Number To Fractional String(number=w347, precision (6)=w337) -> (F-format string=w342:string)  [unwired: 2 in]
            n131 = Number To Fractional String(number=w346, precision (6)=w337) -> (F-format string=w344:string)  [unwired: 2 in]
            n132 = call <userlib>:"DataCell_NbPASSFAIL_Bool.vi"("Tableau en entrée"=w359) -> ("Chaîne"=w357:string, "Chaîne 2"=w358:string)  [unwired: 8 in, 1 out]
            n133 = Number To Decimal String(number=w362) -> (decimal integer string=w370:string)  [unwired: 1 in]
            n134 = call <userlib>:"PASSFAIL.vi"("E"=w341) -> ("S"=w338:string)  [unwired: 10 in]
            n135 = call <userlib>:"PASSFAIL.vi"("E"=w349) -> ("S"=w352:string)  [unwired: 10 in]
            n136 = Build Array(w370, "Communication CAN" ("élément"), w358, w357, "NA" ("élément")) -> (w373:string[])
            n137 = Replace Array Subset(array=string[][] [["Communication CAN", "", "NA", "NA", "", "Communication entre PC et PDU"], ["Courant I(A)", "", "", "", "", "Consommation du courant sur l'alim TENMA 12V"]] ("Tableau"), new element #1=w351, index (row) #1=w356, index (col) #1=1 ("disabled index (col)"), new element #2=w352, index (row) #2=w356, index (col) #2=4 ("disabled index (col)"), new element #3=w348, index (row) #3=w340, index (col) #3=w340, new element #4=w344, index (row) #4=w340, index (col) #4=2 ("disabled index (col)"), new element #5=w342, index (row) #5=w340, index (col) #5=3 ("disabled index (col)"), new element #6=w338, index (row) #6=w340, index (col) #6=4 ("disabled index (col)")) -> (w360:string[][])
            n138 = call "HTML_Table_Head.vi"("entrée d'erreur (pas d'erreur)"=w366, "Tableau"=w373, "chaîne en entrée"=w364) -> ("sortie d'erreur"=w372:errorcluster, "result string"=w371:string)  [unwired: 7 in]
            n139 = call "HTML_Table_Data.vi"("entrée d'erreur (pas d'erreur)"=w372, "Tableau"=w360, "chaîne en entrée"=w371) -> ("sortie d'erreur"=w365:errorcluster, "result string"=w361:string)  [unwired: 7 in]
          }
          frame "OCV" {
            w389 = 0 ("index (row)")
            # "04/11/2022;Test# 3 - Vpack"
            n140 = global read "VG_OCV30max_P.vi" "OCV30max"() -> (w384:dbl)
            n141 = global read "IS30%_P.vi" "VG IS30% ?"() -> (w382:bool)
            n142 = global read "VG_OCV70max_P.vi" "OCV70max"() -> (w383:dbl)
            n143 = global read "VG_OCV30min_P.vi" "OCV30min"() -> (w381:dbl)
            n144 = global read "VG_OCV70min_P.vi" "OCV70min"() -> (w380:dbl)
            n145 = Index Array(array=w407) -> (element #3=w392:string)  [unwired: 3 in, 2 out]
            n146 = Fract/Exp String To Number(string=w392) -> (number=w377:dbl)  [unwired: 3 in, 1 out]
            n147 = Select(t=w381, s=w382, f=w380) -> (s? t:f=w379:dbl)
            n148 = Select(t=w384, s=w382, f=w383) -> (s? t:f=w378:dbl)
            n149 = In Range and Coerce(upper limit=w378, x=w377, lower limit=w379) -> (In Range?=w387:bool)  [unwired: 1 out]
            n150 = Build Array(w387) -> (w399:bool[])
            n151 = Increment(x=w403) -> (x+1=w402:i32)
            n152 = call <userlib>:"DataCell_NbPASSFAIL_Bool.vi"("Tableau en entrée"=w399) -> ("Chaîne"=w397:string, "Chaîne 2"=w398:string)  [unwired: 8 in, 1 out]
            n153 = Number To Decimal String(number=w402) -> (decimal integer string=w410:string)  [unwired: 1 in]
            n154 = call <userlib>:"PASSFAIL.vi"("E"=w387) -> ("S"=w391:string)  [unwired: 10 in]
            n155 = Number To Fractional String(number=w379, precision (6)=i16 2) -> (F-format string=w395:string)  [unwired: 2 in]
            n156 = Number To Fractional String(number=w377, precision (6)=i16 2 ("précision (6)")) -> (F-format string=w376:string)  [unwired: 2 in]
            n157 = Number To Fractional String(number=w378, precision (6)=i16 2) -> (F-format string=w385:string)  [unwired: 2 in]
            n158 = Build Array(w410, "OCV" ("élément"), w398, w397, "NA" ("élément")) -> (w413:string[])
            n159 = Replace Array Subset(array=string[][] [["Tension Pack (V)", "", "", "", "", "Tension du pack"]] ("Tableau"), new element #1=w376, index (row) #1=w389, index (col) #1=1 ("disabled index (col)"), new element #2=w395, index (row) #2=w389, index (col) #2=2 ("disabled index (col)"), new element #3=w385, index (row) #3=w389, index (col) #3=3 ("disabled index (col)"), new element #4=w391, index (row) #4=w389, index (col) #4=4 ("disabled index (col)")) -> (w400:string[][])
            n160 = call "HTML_Table_Head.vi"("entrée d'erreur (pas d'erreur)"=w406, "Tableau"=w413, "chaîne en entrée"=w404) -> ("sortie d'erreur"=w412:errorcluster, "result string"=w411:string)  [unwired: 7 in]
            n161 = call "HTML_Table_Data.vi"("entrée d'erreur (pas d'erreur)"=w412, "Tableau"=w400, "chaîne en entrée"=w411) -> ("sortie d'erreur"=w405:errorcluster, "result string"=w401:string)  [unwired: 7 in]
          }
          frame "IdleCurrent" {
            # "Pourquoi je rajoute 0.001 dans le test \nde comparaison ?\nparceque cette fonction compare si \nle nb est strictement inf/sup"
            # "IdleCurrent;0.1;50?;49.5;100?;99.5;174?;173.6;-50?;-49.0;-100?;-100.1;-174?;-174;CurrentDir;same"
            # "04/11/2022;Test# 3 - Vpack"
            n162 = Index Array(array=w436, index #1=2 ("index")) -> (element #1=w425:string, element #3=w424:string, element #5=w423:string, element #7=w422:string, element #9=w421:string, element #11=w420:string, element #13=w419:string, element #15=w418:string)  [unwired: 14 in, 7 out]
            n163 = Build Array(w425, w424, w423, w422, w421, w420, w419, w418) -> (w417:string[])
            n164 = for {
              tunnel: string[][] [["Courant à vide (A)", "", "0", "0.5", "", "Le courant lorsque le produit est à vide avec contacteurs fermés"], ["Courant à 50A", "", "48.5", "51.5", "", "Le courant mesuré par la PDU (consigne +50A)"], ["Courant à 100A", "", "98.5", "101.5", "", "Le courant mesuré par la PDU (consigne +100A)"], ["Courant à 174A", "", "172.5", "175.5", "", "Le courant mesuré par la PDU (consigne +174A)"], ["Courant à -50A", "", "-51.5", "-48.5", "", "Le courant mesuré par la PDU (consigne -50A)"], ["Courant à -100A", "", "-101.5", "-98.5", "", "Le courant mesuré par la PDU (consigne -100A)"], ["Courant à -174A", "", "-175.5", "-172.5", "", "Le courant mesuré par la PDU (consigne -174A)"], ["Direction du courant", "", "NA", "NA", "", "Verification du sens du courant entre la PDU est l'alimentaion ITECH"]] ("Tableau") -> [w451] mode=indexing
              tunnel: w417 -> [w445] mode=indexing
              tunnel: [w444] -> w426 mode=indexing
              tunnel: [w443] -> w416 mode=indexing
              i -> [w448]
              n165 = Fract/Exp String To Number(string=w445) -> (number=w446:dbl)  [unwired: 3 in, 1 out]
              n166 = case shown="1" w448 {
                tunnel: [w455 w459 w463 w464 w468 w472 w479 w480] -> w443
                tunnel: w446 -> [w452 w456 w460 w465 w469 w473 w476 _]
                tunnel: w445 -> [_ _ _ _ _ _ _ w482]
                frame 0, Default {
                  n167 = In Range and Coerce(upper limit=0.501, x=w452, lower limit=0.0 ("upper limit")) -> (In Range?=w455:bool)  [unwired: 1 out]
                }
                frame 1 {
                  n168 = In Range and Coerce(upper limit=51.501, x=w456, lower limit=48.499 ("upper limit")) -> (In Range?=w459:bool)  [unwired: 1 out]
                }
                frame 2 {
                  n169 = In Range and Coerce(upper limit=101.501, x=w460, lower limit=98.499 ("upper limit")) -> (In Range?=w463:bool)  [unwired: 1 out]
                }
                frame 3 {
                  n170 = In Range and Coerce(upper limit=175.501, x=w465, lower limit=172.499 ("upper limit")) -> (In Range?=w464:bool)  [unwired: 1 out]
                }
                frame 4 {
                  n171 = In Range and Coerce(upper limit=-48.5, x=w469, lower limit=-51.5 ("upper limit")) -> (In Range?=w468:bool)  [unwired: 1 out]
                }
                frame 5 {
                  n172 = In Range and Coerce(upper limit=-98.499, x=w473, lower limit=-101.501 ("upper limit")) -> (In Range?=w472:bool)  [unwired: 1 out]
                }
                frame 6 {
                  n173 = In Range and Coerce(upper limit=-172.499, x=w476, lower limit=-175.501 ("upper limit")) -> (In Range?=w479:bool)  [unwired: 1 out]
                }
                frame 7 {
                  n174 = Equal?(x=w482, y="OK") -> (x = y?=w480:bool)
                }
              }
              n175 = call <userlib>:"PASSFAIL.vi"("E"=w443) -> ("S"=w447:string)  [unwired: 10 in]
              n176 = Replace Array Subset(array=w451, new element #1=w445, index #1=1 ("index"), new element #2=w447, index #2=4 ("index")) -> (w444:string[])
            }
            n177 = Increment(x=w432) -> (x+1=w431:i32)
            n178 = call <userlib>:"DataCell_NbPASSFAIL_Bool.vi"("Tableau en entrée"=w416) -> ("Chaîne"=w428:string, "Chaîne 2"=w429:string)  [unwired: 8 in, 1 out]
            n179 = Number To Decimal String(number=w431) -> (decimal integer string=w439:string)  [unwired: 1 in]
            n180 = Build Array(w439, "Test du courant" ("élément"), w429, w428, "NA" ("élément")) -> (w442:string[])
            n181 = call "HTML_Table_Head.vi"("entrée d'erreur (pas d'erreur)"=w435, "Tableau"=w442, "chaîne en entrée"=w433) -> ("sortie d'erreur"=w441:errorcluster, "result string"=w440:string)  [unwired: 7 in]
            n182 = call "HTML_Table_Data.vi"("entrée d'erreur (pas d'erreur)"=w441, "Tableau"=w426, "chaîne en entrée"=w440) -> ("sortie d'erreur"=w434:errorcluster, "result string"=w430:string)  [unwired: 7 in]
          }
          frame "DataDyn" {
            n183 = call "micro1 pvgen500_P.vi"("FluxStrIn"=w485, "Numin"=w484, "errin"=w491, "Data label"="Données dynamiques" ("testlabel"), "tab ref"=string[][] [["VCell Max (mV)", "", "", "", "", "Tension maximale  des cellules"], ["VCell Min (mV)", "", "", "", "", "Tension minimale  des cellules"], ["NTC Max (°C)", "", "", "", "", "Température maximale"], ["NTC Min (°C)", "", "", "", "", "Température minimale"], ["Delta VCell (mV)", "", "", "", "", "Différence de tensions entre cellules"], ["Delta NTC (°C)", "", "", "", "", "Différence de température entre cellules"], ["SOC", "", "", "", "", "Niveau de tesnion du pack"], ["SOH", "", "", "", "", "L'état de santé de la batterie"]] ("Tableau"), "ligne à traiter"=w487) -> ("result string"=w489:string, "Numout"=w483:i32, "errout"=w490:errorcluster)  [unwired: 11 in]
          }
          frame "DCIR-" {
            w510 = i16 2 ("précision (6)")
            n184 = Index Array(array=w528) -> (element #3=w515:string, element #5=w502:string)  [unwired: 5 in, 3 out]
            n185 = global read "VG_DCIR+OUIouNON_P.vi" "VG_DCIR+ ?"() -> (w507:bool)
            n186 = Fract/Exp String To Number(string=w515) -> (number=w497:dbl)  [unwired: 3 in, 1 out]
            n187 = global read "VG_DCIRmin_P.vi" "DCIRmin"() -> (w494:dbl)
            n188 = Fract/Exp String To Number(string=w502) -> (number=w493:dbl)  [unwired: 3 in, 1 out]
            n189 = global read "VG_DCIRmax_P.vi" "DCIRmax"() -> (w495:dbl)
            n190 = Select(t=i16 2 ("précision (6)"), s=w507, f=i16 1) -> (s? t:f=w504:i16)
            n191 = call <userlib>:"InRange.vi"("min"=w494, "x"=w493, "max"=w495) -> ("In range?"=w492:bool)  [unwired: 1 in]
            n192 = call <userlib>:"InRange.vi"("min"=w494, "x"=w497, "max"=w495) -> ("In range?"=w496:bool)  [unwired: 1 in]
            n193 = global read "VG_DCIR+OUIouNON_P.vi" "VG_DCIR+ ?"() -> (w501:bool)
            n194 = Build Array(w496, w492) -> (w518:bool[])
            n195 = call <userlib>:"PASSFAIL.vi"("E"=w496) -> ("S"=w511:string)  [unwired: 10 in]
            n196 = call <userlib>:"PASSFAIL.vi"("E"=w492) -> ("S"=w503:string)  [unwired: 10 in]
            n197 = call <userlib>:"DataCell_NbPASSFAIL_Bool.vi"("Tableau en entrée"=w518) -> ("Chaîne"=w500:string, "Chaîne 2"=w517:string)  [unwired: 8 in, 1 out]
            n198 = Increment(x=w524) -> (x+1=w521:i32)
            n199 = Number To Fractional String(number=w494, precision (6)=w510) -> (F-format string=w509:string)  [unwired: 2 in]
            n200 = Number To Fractional String(number=w495, precision (6)=w510) -> (F-format string=w508:string)  [unwired: 2 in]
            n201 = Select(t=w500, s=w501, f="0") -> (s? t:f=w499:string)
            n202 = Number To Decimal String(number=w521) -> (decimal integer string=w523:string)  [unwired: 1 in]
            n203 = for {
              N: w504 -> [_]
              tunnel: [string[] ["DCIR- (mOhm)", "", "", "", "", "Résistance interne à une décharge de -174A"] ("Tableau")] -> w529 mode=indexing
            }
            n204 = Build Array(w523, "DCIR" ("élément"), w517, w499, "NA" ("élément")) -> (w520:string[])
            n205 = call "HTML_Table_Head.vi"("entrée d'erreur (pas d'erreur)"=w525, "Tableau"=w520, "chaîne en entrée"=w519) -> ("sortie d'erreur"=w527:errorcluster, "result string"=w514:string)  [unwired: 7 in]
            n206 = for {
              tunnel: w529 -> [w540] mode=indexing
              tunnel: w515 -> [w535]
              tunnel: [w539] -> w513 mode=indexing
              tunnel: w511 -> [w532]
              tunnel: w509 -> [w534]
              tunnel: w508 -> [w533]
              tunnel: w502 -> [w531]
              tunnel: w503 -> [w530]
              i -> [w538]
              n207 = Greater?(x=w538, y=0) -> (0:w536:bool)
              n208 = case shown="True" w536 {
                tunnel: w540 -> [w550 w562]
                tunnel: [w549 w551] -> w539
                tunnel: w535 -> [w547 _]
                tunnel: w534 -> [w545 w556]
                tunnel: w533 -> [w543 w554]
                tunnel: w532 -> [w542 _]
                tunnel: w531 -> [_ w558]
                tunnel: w530 -> [_ w552]
                frame False {
                  n209 = Replace Array Subset(array=w550, new element #1=w547, index #1=1 ("index"), new element #2=w545, index #2=2 ("index"), new element #3=w543, index #3=3 ("index"), new element #4=w542, index #4=4 ("index")) -> (w549:string[])
                }
                frame True {
                  n210 = Replace Array Subset(array=w562, new element #1="DCIR- (mOhm)" ("new element/subarray"), index #1=0 ("index"), new element #2=w558, index #2=1 ("index"), new element #3=w556, index #3=2 ("index"), new element #4=w554, index #4=3 ("index"), new element #5=w552, index #5=4 ("index")) -> (w551:string[])
                }
              }
            }
            n211 = call "HTML_Table_Data.vi"("entrée d'erreur (pas d'erreur)"=w527, "Tableau"=w513, "chaîne en entrée"=w514) -> ("sortie d'erreur"=w526:errorcluster, "result string"=w512:string)  [unwired: 7 in]
          }
          frame "DTC" {
            w575 = 0 ("indice (ligne)")
            n212 = Index Array(array=w579) -> (element #3=w568:string)  [unwired: 3 in, 2 out]
            n213 = Equal?(x=w568, y="NO DTC") -> (x = y?=w567:bool)
            n214 = Build Array(w567) -> (w586:bool[])
            n215 = call <userlib>:"DataCell_NbPASSFAIL_Bool.vi"("Tableau en entrée"=w586) -> ("Chaîne"=w584:string, "Chaîne 2"=w585:string)  [unwired: 8 in, 1 out]
            n216 = call <userlib>:"PASSFAIL.vi"("E"=w567) -> ("S"=w566:string)  [unwired: 10 in]
            n217 = Increment(x=w582) -> (x+1=w564:i32)
            n218 = Number To Decimal String(number=w564) -> (decimal integer string=w588:string)  [unwired: 1 in]
            n219 = Build Array(w588, "DTC" ("élément"), w585, w584, "NA" ("élément")) -> (w581:string[])
            n220 = call "HTML_Table_Head.vi"("entrée d'erreur (pas d'erreur)"=w589, "Tableau"=w581, "chaîne en entrée"=w580) -> ("sortie d'erreur"=w592:errorcluster, "result string"=w591:string)  [unwired: 7 in]
            n221 = Replace Array Subset(array=string[][] [["DTC", "", "", "", "", "Abscence de code d'erreur remonter pas le système"]] ("Tableau"), new element #1=w568, index (row) #1=w575, index (col) #1=1 ("indice désactivé (col)"), new element #2="NA" ("nouvel élément/sous-tableau"), index (row) #2=w575, index (col) #2=2 ("indice désactivé (col)"), new element #3="NA" ("nouvel élément/sous-tableau"), index (row) #3=w575, index (col) #3=3 ("indice désactivé (col)"), new element #4=w566, index (row) #4=w575, index (col) #4=4 ("indice désactivé (col)")) -> (w577:string[][])
            n222 = call "HTML_Table_Data.vi"("entrée d'erreur (pas d'erreur)"=w592, "Tableau"=w577, "chaîne en entrée"=w591) -> ("sortie d'erreur"=w590:errorcluster, "result string"=w578:string)  [unwired: 7 in]
          }
          frame "FinalOCV" {
            w595 = 0 ("index (row)")
            w594 = 4 ("indice désactivé (col)")
            w599 = 1 ("indice (ligne)")
            # "ocv final\nest tjs pass"
            n223 = Index Array(array=w608) -> (element #3=w596:string, element #5=w597:string)  [unwired: 5 in, 3 out]
            n224 = Fract/Exp String To Number(string=w597) -> (number=w602:dbl)  [unwired: 3 in, 1 out]
            n225 = Equal To 0?(x=w602) -> (x = 0?=w601:bool)
            n226 = Build Array(w601) -> (w615:bool[])
            n227 = call <userlib>:"DataCell_NbPASSFAIL_Bool.vi"("Tableau en entrée"=w615) -> ("Chaîne"=w613:string, "Chaîne 2"=w614:string)  [unwired: 8 in, 1 out]
            n228 = call <userlib>:"PASSFAIL.vi"("E"=w601) -> ("S"=w600:string)  [unwired: 10 in]
            n229 = Increment(x=w611) -> (x+1=w603:i32)
            n230 = Number To Decimal String(number=w603) -> (decimal integer string=w617:string)  [unwired: 1 in]
            n231 = Build Array(w617, "Tension en OFF" ("élément"), w614, w613, "NA" ("élément")) -> (w610:string[])
            n232 = call "HTML_Table_Head.vi"("entrée d'erreur (pas d'erreur)"=w618, "Tableau"=w610, "chaîne en entrée"=w609) -> ("sortie d'erreur"=w621:errorcluster, "result string"=w620:string)  [unwired: 7 in]
            n233 = call <userlib>:"PASSFAIL.vi"("E"=TRUE) -> ("S"=w593:string)  [unwired: 10 in]
            n234 = Replace Array Subset(array=string[][] [["OCV Final", "", "NA", "NA", "", "Tension pack avant livraison "], ["Tension en mode Off", "", "0", "0", "", "Verification de l'absence de tension et que les contacteurs sont bien ouverts"]] ("Tableau"), new element #1=w596, index (row) #1=w595, index (col) #1=w599, new element #2=w597, index (row) #2=w599, index (col) #2=1 ("indice désactivé (col)"), new element #3=w600, index (row) #3=w599, index (col) #3=w594, new element #4=w593, index (row) #4=w595, index (col) #4=w594) -> (w606:string[][])
            n235 = call "HTML_Table_Data.vi"("entrée d'erreur (pas d'erreur)"=w621, "Tableau"=w606, "chaîne en entrée"=w620) -> ("sortie d'erreur"=w619:errorcluster, "result string"=w607:string)  [unwired: 7 in]
          }
        }
      }
    }
  }
  n236 = Concatenate Strings(w12, "\\" ("chaîne"), w10) -> (w9:string)
  n237 = String To Path(string=w9) -> (path=w15:path)
  "network out" <- w15
  n238 = Search and Replace String(replace all?=TRUE ("tout remplacer ? (F)"), input string=w49, search string="<td class=\"core1 testpass\">FAIL</td>" ("chaîne recherchée"), replace string="<td class=\"core1 testfail\">FAIL</td>" ("chaîne de remplacement (\"\")"), error in=w47) -> (result string=w33:string, number of replacements=w28:i32, error out=w44:errorcluster)  [unwired: 3 in, 1 out]
  n239 = Search and Replace String(replace all?=TRUE ("tout remplacer ? (F)"), input string=w33, search string="<td class=\"core1 testpass\">PASS</td>" ("chaîne recherchée"), error in=w44) -> (number of replacements=w36:i32, error out=w40:errorcluster)  [unwired: 4 in, 2 out]
  "nombre de remplacements" <- w36
  n240 = Number To Decimal String(number=w36) -> (decimal integer string=w35:string)  [unwired: 1 in]
  n241 = Number To Decimal String(number=w28) -> (decimal integer string=w34:string)  [unwired: 1 in]
  n242 = Search and Replace String(input string=w33, search string="<!--NBTESTOK-->" ("chaîne recherchée"), replace string=w35, error in=w40) -> (result string=w41:string, error out=w39:errorcluster)  [unwired: 4 in, 2 out]
  n243 = Equal To 0?(x=w28) -> (x = 0?=w20:bool)
  n244 = Search and Replace String(input string=w41, search string="<!--NBTESTKO-->" ("chaîne recherchée"), replace string=w34, error in=w39) -> (result string=w23:string, error out=w27:errorcluster)  [unwired: 4 in, 2 out]
  n245 = Search and Replace String(input string=w23, search string="Résultat du test :\t</td><td class=\"resume5\" colspan=\"3\"><div><span style=\"float:left\" id=\"result\"><font size = \"5pt\" color=\"green\"><b>CONFORME</b>", replace string="Résultat du test :\t</td><td class=\"resume5\" colspan=\"3\"><div><span style=\"float:left\" id=\"result\"><font  size = \"5pt\" color=\"red\"><b>NON CONFORME</b>", error in=w27) -> (result string=w5:string, error out=w26:errorcluster)  [unwired: 4 in, 2 out]
  n246 = Search and Replace String(input string=w5, search string=".resume1,.resume3,.resume4,.resume5,.resume6,.resume7{background-color:#e6feef;padding:7px;border:1px solid black;}\n.resume0{border:1px solid black;background-color:#e6feef;font-weight: bold;padding:0px;text-align: center;}", replace string=".resume1,.resume3,.resume4,.resume5,.resume6,.resume7{background-color:#fdebd0;padding:7px;border:1px solid black;}\n.resume0{border:1px solid black;background-color:#fdebd0;font-weight: bold;padding:0px;text-align: center;}") -> (result string=w4:string)  [unwired: 5 in, 3 out]
  n247 = Select(t=w23, s=w20, f=w4) -> (s? t:f=w24:string)
  "Chaîne" <- w24
  n248 = Not Equal?(x=w15, y=path "") -> (x != y?=w17:bool)
  n249 = Open/Create/Replace File(file path (use dialog)=w50, error in=w26, operation (0:open)=w32) -> (refnum out=w56:refnum<file>, error out=w58:errorcluster)  [unwired: 3 in, 1 out]
  n250 = case shown="True" w17 {
    tunnel: w32 -> [_ w627]
    tunnel: w15 -> [_ w626]
    tunnel: w26 -> [_ w625]
    tunnel: w24 -> [_ w624]
    tunnel: [errorcluster {"status"=FALSE, "code"=0, "source"=""} ("error out") w623] -> w22
    frame False {
    }
    frame True {
      n251 = Open/Create/Replace File(file path (use dialog)=w626, error in=w625, operation (0:open)=w627) -> (refnum out=w628:refnum<file>, error out=w630:errorcluster)  [unwired: 3 in, 1 out]
      n252 = Write to Text File(file (use dialog)=w628, text=w624, error in=w630) -> (refnum out=w629:refnum<file>, error out=w631:errorcluster)  [unwired: 1 in, 1 out]
      n253 = Close File(refnum=w629, error in=w631) -> (error out=w623:errorcluster)  [unwired: 1 out]
    }
  }
  n254 = Write to Text File(file (use dialog)=w56, text=w24, error in=w58) -> (refnum out=w57:refnum<file>, error out=w59:errorcluster)  [unwired: 1 in, 1 out]
  n255 = Close File(refnum=w57, error in=w59) -> (error out=w21:errorcluster)  [unwired: 1 out]
  n256 = Merge Errors(w21, w22) -> (w19:errorcluster)
  "sortie d'erreur" <- w19
  n257 = Compound Arithmetic op=AND ("Opérateur arithmétique")(w20, invert w19) -> (→"tout bon":bool)
